vi "Three part faster sub live.vi"() -> ()   [LabVIEW 2009]
uses:
  <vilib>/vision/NI_Vision_Development_Module.lvlib
  <vilib>/Instr/_visa.llb/VISA Configure Serial Port (Instr).vi
  <vilib>/vision/driver/NI_Vision_Acquisition_Software.lvlib
  <vilib>/vision/Image Controls.llb/IMAQ Image.ctl
  <vilib>/userDefined/High Color/IMAQdx.ctl
panel:
  out "Drum Cluster":T1
  out "Guitar Cluster":T2
  out "Bass Cluster":T3
  in  "Camera":T4="cam0"
  in  "Orange Bass":T5={"Global Rectangle"=[220, 302, 227, 392], "Contours"=[{"ID"=enum."External", "Type"=2, "Coordinates"=[226, 391, 220, 302]}]} {"Contours"."Type" items=["No Selection", "Point", "Line", "Rectangle", "Oval", "Polygon", "Freehand Region", "Annulus", "Unused2", "Unused3", "Broken Line", "Freehand Line", "Rotated Rectangle"]}
  in  "Blue Bass":T5={"Global Rectangle"=[192, 292, 199, 386], "Contours"=[{"ID"=enum."External", "Type"=2, "Coordinates"=[192, 385, 198, 292]}]} {"Contours"."Type" items=["No Selection", "Point", "Line", "Rectangle", "Oval", "Polygon", "Freehand Region", "Annulus", "Unused2", "Unused3", "Broken Line", "Freehand Line", "Rotated Rectangle"]}
  in  "playtime":dbl=90.0
  out "decimal integer string 2":string
  out "number 2":u32
  in  "Orange Guitar":T5={"Global Rectangle"=[587, 282, 628, 378], "Contours"=[{"ID"=enum."External", "Type"=2, "Coordinates"=[627, 377, 587, 282]}]} {"Contours"."Type" items=["No Selection", "Point", "Line", "Rectangle", "Oval", "Polygon", "Freehand Region", "Annulus", "Unused2", "Unused3", "Broken Line", "Freehand Line", "Rotated Rectangle"]}
  in  "Yellow Guitar":T5={"Global Rectangle"=[546, 282, 563, 376], "Contours"=[{"ID"=enum."External", "Type"=2, "Coordinates"=[562, 375, 546, 282]}]} {"Contours"."Type" items=["No Selection", "Point", "Line", "Rectangle", "Oval", "Polygon", "Freehand Region", "Annulus", "Unused2", "Unused3", "Broken Line", "Freehand Line", "Rotated Rectangle"]}
  in  "Green Guitar":T5={"Global Rectangle"=[498, 284, 505, 376], "Contours"=[{"ID"=enum."External", "Type"=2, "Coordinates"=[498, 375, 504, 284]}]} {"Contours"."Type" items=["No Selection", "Point", "Line", "Rectangle", "Oval", "Polygon", "Freehand Region", "Annulus", "Unused2", "Unused3", "Broken Line", "Freehand Line", "Rotated Rectangle"]}
  in  "Blue Guitar":T5={"Global Rectangle"=[569, 290, 594, 372], "Contours"=[{"ID"=enum."External", "Type"=2, "Coordinates"=[593, 371, 569, 290]}]} {"Contours"."Type" items=["No Selection", "Point", "Line", "Rectangle", "Oval", "Polygon", "Freehand Region", "Annulus", "Unused2", "Unused3", "Broken Line", "Freehand Line", "Rotated Rectangle"]}
  in  "Red Guitar":T5={"Global Rectangle"=[526, 284, 530, 370], "Contours"=[{"ID"=enum."External", "Type"=2, "Coordinates"=[529, 369, 526, 284]}]} {"Contours"."Type" items=["No Selection", "Point", "Line", "Rectangle", "Oval", "Polygon", "Freehand Region", "Annulus", "Unused2", "Unused3", "Broken Line", "Freehand Line", "Rotated Rectangle"]}
  in  "Green Bass":T5={"Global Rectangle"=[100, 292, 131, 371], "Contours"=[{"ID"=enum."External", "Type"=2, "Coordinates"=[100, 370, 130, 292]}]} {"Contours"."Type" items=["No Selection", "Point", "Line", "Rectangle", "Oval", "Polygon", "Freehand Region", "Annulus", "Unused2", "Unused3", "Broken Line", "Freehand Line", "Rotated Rectangle"]}
  in  "Red Bass":T5={"Global Rectangle"=[129, 294, 154, 376], "Contours"=[{"ID"=enum."External", "Type"=2, "Coordinates"=[129, 375, 153, 294]}]} {"Contours"."Type" items=["No Selection", "Point", "Line", "Rectangle", "Oval", "Polygon", "Freehand Region", "Annulus", "Unused2", "Unused3", "Broken Line", "Freehand Line", "Rotated Rectangle"]}
  in  "Yellow Bass":T5={"Global Rectangle"=[160, 295, 175, 378], "Contours"=[{"ID"=enum."External", "Type"=2, "Coordinates"=[160, 377, 174, 295]}]} {"Contours"."Type" items=["No Selection", "Point", "Line", "Rectangle", "Oval", "Polygon", "Freehand Region", "Annulus", "Unused2", "Unused3", "Broken Line", "Freehand Line", "Rotated Rectangle"]}
  in  "Mask":T5 {"Contours"."Type" items=["No Selection", "Point", "Line", "Rectangle", "Oval", "Polygon", "Freehand Region", "Annulus", "Unused2", "Unused3", "Broken Line", "Freehand Line", "Rotated Rectangle"]}
  in  "Red Line":T5={"Global Rectangle"=[300, 297, 320, 380], "Contours"=[{"ID"=enum."External", "Type"=2, "Coordinates"=[300, 379, 319, 297]}]} {"Contours"."Type" items=["No Selection", "Point", "Line", "Rectangle", "Oval", "Polygon", "Freehand Region", "Annulus", "Unused2", "Unused3", "Broken Line", "Freehand Line", "Rotated Rectangle"]}
  in  "Blue Line":T5={"Global Rectangle"=[374, 278, 383, 377], "Contours"=[{"ID"=enum."External", "Type"=2, "Coordinates"=[382, 376, 374, 278]}]} {"Contours"."Type" items=["No Selection", "Point", "Line", "Rectangle", "Oval", "Polygon", "Freehand Region", "Annulus", "Unused2", "Unused3", "Broken Line", "Freehand Line", "Rotated Rectangle"]}
  in  "Green Line":T5={"Global Rectangle"=[406, 309, 423, 383], "Contours"=[{"ID"=enum."External", "Type"=2, "Coordinates"=[422, 382, 406, 309]}]} {"Contours"."Type" items=["No Selection", "Point", "Line", "Rectangle", "Oval", "Polygon", "Freehand Region", "Annulus", "Unused2", "Unused3", "Broken Line", "Freehand Line", "Rotated Rectangle"]}
  in  "Yellow Line":T5={"Global Rectangle"=[342, 292, 349, 377], "Contours"=[{"ID"=enum."External", "Type"=2, "Coordinates"=[342, 376, 348, 292]}]} {"Contours"."Type" items=["No Selection", "Point", "Line", "Rectangle", "Oval", "Polygon", "Freehand Region", "Annulus", "Unused2", "Unused3", "Broken Line", "Freehand Line", "Rotated Rectangle"]}
  in  "VISA resource name":refnum<visa-resource-name>
  out "number":u32
  out "decimal integer string":string
  out "Image Dst Out":T6
  in  "stop":bool
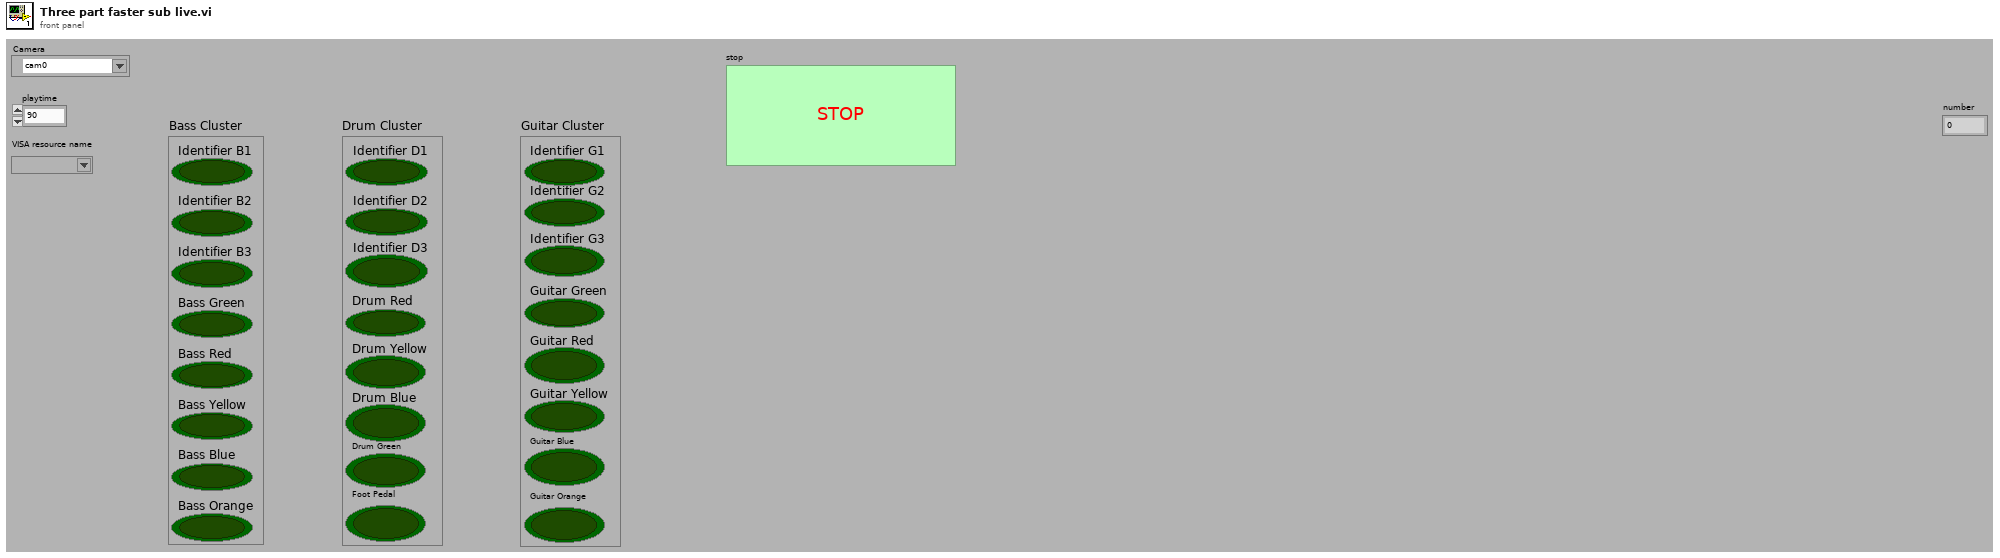
[diagram p1: front panel]
types:
  T1 = cluster{"Identifier D1":bool, "Identifier D2":bool, "Identifier D3":bool, "Drum Red":bool, "Drum Yellow":bool, "Drum Blue":bool, "Drum Green":bool, "Foot Pedal":bool}
  T2 = cluster{"Identifier G1":bool, "Identifier G2":bool, "Identifier G3":bool, "Guitar Green":bool, "Guitar Red":bool, "Guitar Yellow":bool, "Guitar Blue":bool, "Guitar Orange":bool}
  T3 = cluster{"Identifier B1":bool, "Identifier B2":bool, "Identifier B3":bool, "Bass Green":bool, "Bass Red":bool, "Bass Yellow":bool, "Bass Blue ":bool, "Bass Orange":bool}
  T4 = typedef "IMAQdx.ctl" = refnum<k21>
  T5 = cluster{"Global Rectangle":i32[], "Contours":cluster{"ID":enum32{"External", "Internal"}, "Type":u32, "Coordinates":i32[]}[]}
  T6 = typedef "IMAQ Image.ctl" = refnum<image>
  T7 = typedef "Image Type" = u32
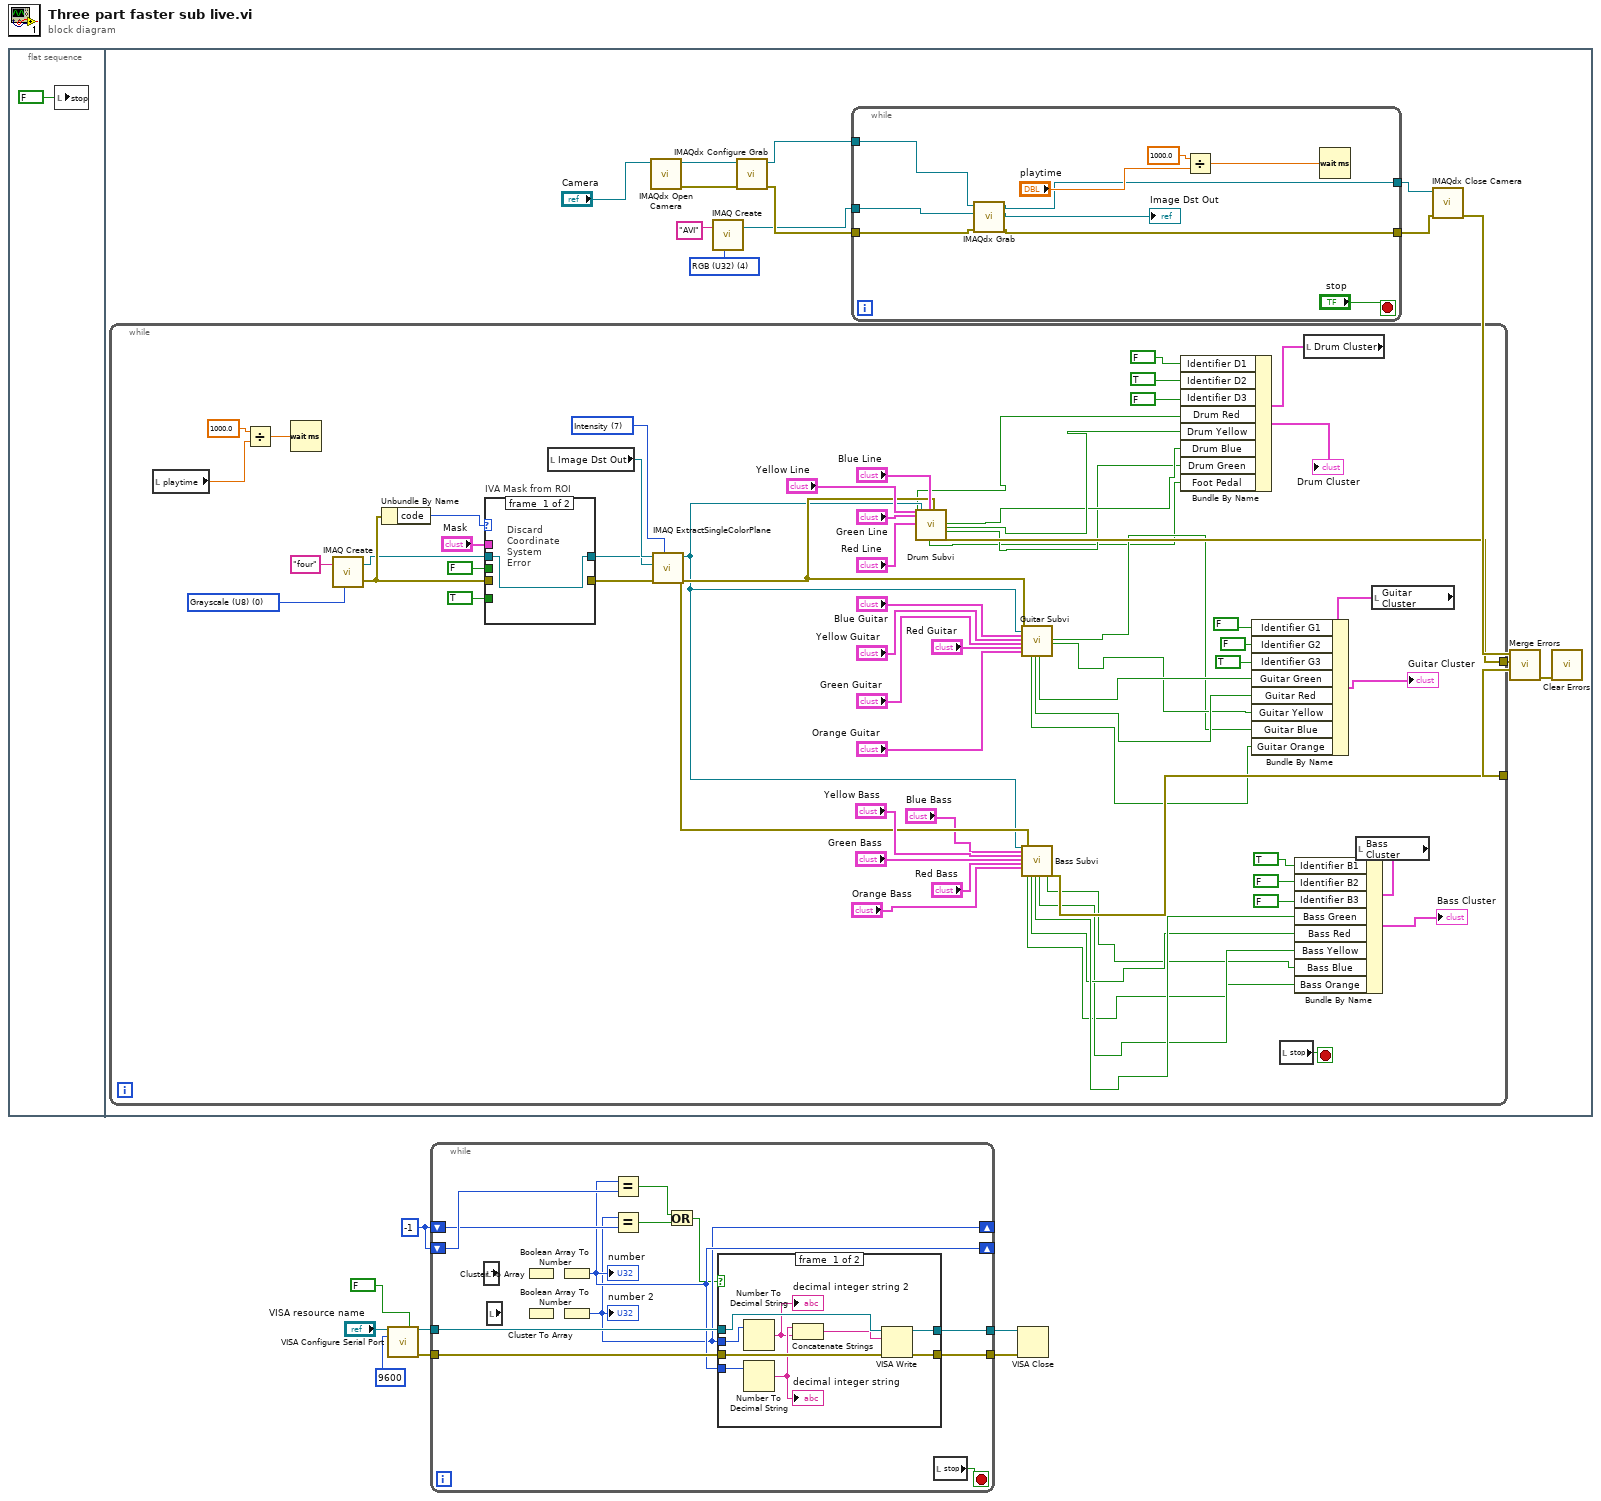
[diagram p0: block diagram]
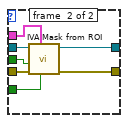
[diagram p3: hidden frame]
diagram:
  w1 = -1
  n1 = flat-sequence {
    frame #0 {
      n2 = local write "stop"(FALSE ("stop")) -> ()
    }
    frame #1 {
      w20 = T7 4 items=["Grayscale (U8)", "Grayscale (I16)", "Grayscale (SGL)", "Complex (CSG)", "RGB (U32)", "HSL (U32)", "RGB (U64)", "Grayscale (U16)"] ("Image Type")
      n3 = while {
        tunnel: [w72] -> w22
        tunnel: [w64] -> w21
        stop <- w86 stop-if-true
        w82 = T7 0 items=["Grayscale (U8)", "Grayscale (I16)", "Grayscale (SGL)", "Complex (CSG)", "RGB (U32)", "HSL (U32)", "RGB (U64)", "Grayscale (U16)"] ("Image Type")
        w87 = 7 items=["Red", "Green", "Blue", "Hue", "Saturation", "Luminance", "Value", "Intensity"] ("Color Plane")
        n4 = local read "playtime"() -> (w56:dbl)
        n5 = Divide(x=1000.0, y=w56) -> (x/y=w85:dbl)
        n6 = Wait (ms)(milliseconds to wait=w85) -> ()  [unwired: 1 out]
        n7 = call "IMAQ Create"("Image Name"="four", "Image Type"=w82) -> ("New Image"=w75:T6, "error out"=w76:errorcluster)  [unwired: 3 in]
        n8 = Unbundle By Name(w76) -> ("code"=w80:i32)
        n9 = case "IVA Mask from ROI" shown="Default" w80 {
          tunnel: "Mask" -> [_ w95]
          tunnel: TRUE ("Shrink") -> [_ w94]
          tunnel: w75 -> [w88 w93]
          tunnel: w76 -> [_ w92]
          tunnel: [_ w91] -> w77
          tunnel: [w88 w90] -> w73
          tunnel: FALSE ("Out / In") -> [_ w89]
          frame #0 {
            # "Discard\nCoordinate\nSystem\nError"
          }
          frame #1 {
            n10 = call <vilib>:"IVA Mask from ROI.vi"("Shrink"=w94, "ROI Descriptor"=w95, "error in (no error)"=w92, "Out / In"=w89, "Image Src"=w93) -> ("error out"=w91:errorcluster, "Image Out"=w90:T6)  [unwired: 5 out]
          }
        }
        n11 = local read "Image Dst Out"() -> (w83:T6)
        n12 = call "IMAQ ExtractSingleColorPlane"("Color Plane"=w87, "error in (no error)"=w77, "Image Dst"=w73, "Image Src"=w83) -> ("error out"=w63:errorcluster, "Image Dst Out"=w58:T6)  [unwired: 6 out]
        n13 = call "Drum Subvi.vi"("Yellow Line"="Yellow Line", "Green Line"="Green Line", "Red Line"="Red Line", "Image Dst Out"=w58, "Blue Line"="Blue Line", "error out"=w63) -> ("LED Red"=w28:bool, "Foot Pedal"=w24:bool, "Blue Drum 2"=w26:bool, "Yellow Drum"=w27:bool, "Green Drum"=w25:bool, "error out 2"=w72:errorcluster)  [unwired: 12 in, 4 out]
        n14 = call "Guitar Subvi.vi"("error out"=w63, "Image Dst Out"=w58, "Blue Guitar 2"="Blue Guitar", "Yellow Guitar 2"="Yellow Guitar", "Green Guitar 2"="Green Guitar", "Red Guitar 2"="Red Guitar", "Orange Guitar 2"="Orange Guitar") -> ("Orange Guitar LED"=w34:bool, "Red Guitar LED"=w37:bool, "Green Guitar LED"=w38:bool, "Blue Guitar LED"=w35:bool, "Yellow Guitar LED"=w36:bool)  [unwired: 16 in]
        n15 = call "Bass Subvi.vi"("Image Dst Out"=w58, "Blue Bass 2"="Blue Bass", "Yellow Bass 2"="Yellow Bass", "Green Bass 2"="Green Bass", "Red Bass 2"="Red Bass", "Orange Bass 2"="Orange Bass", "error out"=w63) -> ("Orange Bass LED"=w44:bool, "Red Bass LED"=w47:bool, "Green Bass LED"=w48:bool, "Yellow Bass LED"=w46:bool, "Blue Bass LED"=w45:bool, "error out 2"=w64:errorcluster)  [unwired: 15 in]
        n16 = local read "stop"() -> (w86:bool)
        n17 = local read "Drum Cluster"() -> (w32:T1)
        n18 = Bundle By Name(cluster=w32, "Identifier D1"=FALSE, "Identifier D2"=TRUE ("element"), "Identifier D3"=FALSE ("element"), "Drum Red"=w28, "Drum Yellow"=w27, "Drum Blue"=w26, "Drum Green"=w25, "Foot Pedal"=w24) -> (→"Drum Cluster":T1)
        n19 = local read "Bass Cluster"() -> (w53:T3)
        n20 = Bundle By Name(cluster=w53, "Identifier B1"=TRUE, "Identifier B2"=FALSE ("element"), "Identifier B3"=FALSE ("element"), "Bass Green"=w48, "Bass Red"=w47, "Bass Yellow"=w46, "Bass Blue"=w45, "Bass Orange"=w44) -> (→"Bass Cluster":T3)
        n21 = local read "Guitar Cluster"() -> (w42:T2)
        n22 = Bundle By Name(cluster=w42, "Identifier G1"=FALSE ("element"), "Identifier G2"=FALSE ("element"), "Identifier G3"=TRUE ("element"), "Guitar Green"=w38, "Guitar Red"=w37, "Guitar Yellow"=w36, "Guitar Blue"=w35, "Guitar Orange"=w34) -> (→"Guitar Cluster":T2)
      }
      n23 = call <vilib>:"IMAQdx Open Camera.vi"("Session In"="Camera") -> ("error out"=w18:errorcluster, "Session Out"=w17:T4)  [unwired: 9 in]
      n24 = call "IMAQ Create"("Image Name"="AVI", "Image Type"=w20) -> ("New Image"=w13:T6)  [unwired: 3 in, 1 out]
      n25 = call <vilib>:"IMAQdx Configure Grab.vi"("error in"=w18, "Session In"=w17) -> ("error out"=w14:errorcluster, "Session Out"=w15:T4)  [unwired: 8 in]
      n26 = while {
        tunnel: w13 -> [w99]
        tunnel: w14 -> [w101]
        tunnel: [w98] -> w10
        tunnel: [w96] -> w12
        tunnel: w15 -> [w100]
        stop <- "stop" stop-if-true
        n27 = call <vilib>:"IMAQdx Grab.vi"("error in"=w101, "Image In"=w99, "Session In"=w100) -> ("error out"=w96:errorcluster, "Image Out"=→"Image Dst Out":T6, "Session Out"=w98:T4)  [unwired: 5 in, 1 out]
        n28 = Divide(x=1000.0, y="playtime") -> (x/y=w104:dbl)
        n29 = Wait (ms)(milliseconds to wait=w104) -> ()  [unwired: 1 out]
      }
      n30 = call <vilib>:"IMAQdx Close Camera.vi"("error in"=w12, "Session In"=w10) -> ("error out"=w11:errorcluster)  [unwired: 9 in]
      n31 = call <vilib>:"Merge Errors.vi"("error in 3 (no error)"=w21, "error in 2 (no error)"=w22, "error in 1 (no error)"=w11) -> ("error out"=w23:errorcluster)  [unwired: 4 in]
      n32 = call <vilib>:"Clear Errors.vi"("error in (no error)"=w23) -> ()  [unwired: 6 in, 1 out]
    }
  }
  n33 = call-poly "VISA Configure Serial Port"("VISA resource name"="VISA resource name", "Enable Termination\nChar (T)"=FALSE ("Enable Termination\nChar (T)"), "baud rate (9600)"=u32 9600) -> ("VISA resource name out"=w8:refnum<visa-resource-name>, "error out"=w3:errorcluster)  [unwired: 11 in]
  n34 = while {
    shift-right: [w110] -> _
    shift-left: w1 -> [w117]
    tunnel: w8 -> [w116]
    tunnel: [w115] -> w7
    tunnel: w3 -> [w114]
    tunnel: [w113] -> w2
    shift-right: [w109] -> _
    shift-left: w1 -> [w111]
    stop <- w112 stop-if-true
    n35 = local read item#-1() -> ()  [unwired: 1 out]
    n36 = local read item#-1() -> ()  [unwired: 1 out]
    n37 = Cluster To Array() -> ()  [unwired: 1 in, 1 out]
    n38 = Cluster To Array() -> ()  [unwired: 1 in, 1 out]
    n39 = Boolean Array To Number() -> (number=w110:u32)  [unwired: 1 in]
    "number" <- w110
    n40 = Boolean Array To Number() -> (number=w109:u32)  [unwired: 1 in]
    "number 2" <- w109
    n41 = Equal?(x=w110, y=w117) -> (x = y?=w108:bool)
    n42 = Equal?(x=w109, y=w111) -> (x = y?=w107:bool)
    n43 = Or(x=w108, y=w107) -> (x .or. y?=w106:bool)
    n44 = case shown="False" w106 {
      tunnel: w116 -> [w126 w128]
      tunnel: [w125 w128] -> w115
      tunnel: w110 -> [w124 _]
      tunnel: w114 -> [w123 w127]
      tunnel: [w122 w127] -> w113
      tunnel: w109 -> [w121 _]
      frame #0 {
        n45 = Number To Decimal String(number=w121) -> (decimal integer string=w119:string)  [unwired: 1 in]
        "decimal integer string 2" <- w119
        n46 = Number To Decimal String(number=w124) -> (decimal integer string=w120:string)  [unwired: 1 in]
        "decimal integer string" <- w120
        n47 = Concatenate Strings(w120, w119) -> (w118:string)
        n48 = VISA Write(VISA resource name=w126, write buffer=w118, error in (no error)=w123) -> (VISA resource name out=w125:refnum<visa-resource-name>, error out=w122:errorcluster)  [unwired: 1 out]
      }
      frame #1 {
      }
    }
    n49 = local read "stop"() -> (w112:bool)
  }
  n50 = VISA Close(VISA resource name=w7, error in (no error)=w2) -> ()  [unwired: 1 out]
